vi "mhk Basic Acquisition  (no header).vi"() -> ()   [LabVIEW 2010]
uses:
  <vilib>/Utility/error.llb/DialogType.ctl
  <vilib>/DAQmx/read.llb/DAQmx Read (Analog 1D Wfm NChan NSamp).vi
  <vilib>/DAQmx/create/channels.llb/DAQmx Create Channel (AI-Voltage-Basic).vi
  <vilib>/DAQmx/configure/timing.llb/DAQmx Timing (Sample Clock).vi
  Instance          10 42Saved   mhk Basic Acquisition  (no header) .vi
  <vilib>/daqmx/miscellaneous.llb/DAQmx Fill In Error Info.vi
panel:
  in  "Prompt to Save Data?":bool caption="Enable"
  in  "Maximum Value":dbl=5.0 format="%0.2f"
  in  "Minimum Value":dbl=-5.0 format="%0.2f"
  in  "Physical Channel":tag="Dev2/ai0:1"
  in  "Rate":dbl=1000.0 caption="Sample Rate (Hz)" format="%0.2f"
  in  "Samples per Channel":i32=1000
  out "Measurement":waveform(dbl)[](graph)=[{"t0"=timestamp(3384461688.008659 s since 1904-01-01), "dt"=0.001, "Y"=array[1000 elements], "attributes"=variant("NI_ChannelName"=variant(string "Dev2/ai0"), "NI_UnitDescription"=variant(string "Volts"))}, {"t0"=timestamp(3384461688.0086718 s since 1904-01-01), "dt"=0.001, "Y"=array[1000 elements], "attributes"=variant("NI_ChannelName"=variant(string "Dev2/ai1"), "NI_UnitDescription"=variant(string "Volts"))}]
  # "Channel Parameters"
  # "Timing Parameters"
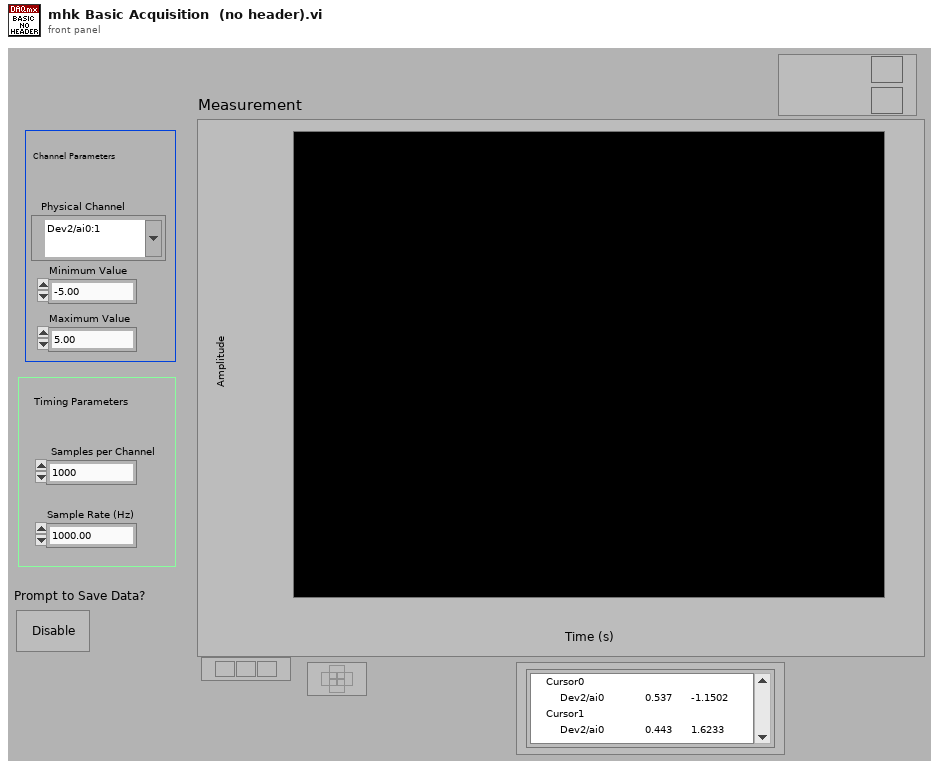
[diagram p1: front panel]
types:
  T1 = typedef "DialogType.ctl" = u16
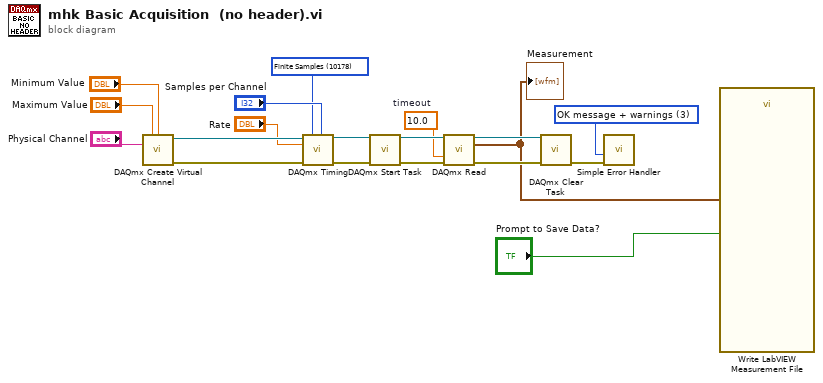
[diagram p0: block diagram]
diagram:
  w4 = T1 3 items=["no dialog", "OK message", "continue or stop message", "OK message + warnings", "continue/stop + warnings"] ("type of dialog (OK msg:1)")
  w5 = 10.0  # timeout
  w9 = 10178 items=["Finite Samples"=10178, "Continuous Samples"=10123] ("sample mode")
  n1 = call-poly <vilib>:"DAQmx Create Virtual Channel.vi"("maximum value"="Maximum Value", "minimum value"="Minimum Value", "physical channels"="Physical Channel") -> ("task out"=w13:refnum<k21>, "error out"=w17:errorcluster)  [unwired: 11 in]
  n2 = call-poly <vilib>:"DAQmx Timing.vi"("task/channels in"=w13, "sample mode"=w9, "samples per channel"="Samples per Channel", "rate"="Rate", "error in"=w17) -> ("task out"=w8:refnum<k21>, "error out"=w7:errorcluster)  [unwired: 9 in]
  n3 = call <vilib>:"DAQmx Start Task.vi"("task/channels in"=w8, "error in"=w7) -> ("task out"=w12:refnum<k21>, "error out"=w16:errorcluster)  [unwired: 12 in]
  n4 = call-poly <vilib>:"DAQmx Read.vi"("task/channels in"=w12, "timeout"=w5, "error in"=w16) -> ("task out"=w11:refnum<k21>, "data"=w2:waveform(dbl)[], "error out"=w6:errorcluster)  [unwired: 10 in]
  "Measurement" <- w2
  n5 = call <vilib>:"DAQmx Clear Task.vi"("task in"=w11, "error in"=w6) -> ("error out"=w14:errorcluster)  [unwired: 13 in]
  n6 = call <vilib>:"Simple Error Handler.vi"("type of dialog (OK msg:1)"=w4, "error in (no error)"=w14) -> ()  [unwired: 3 in, 5 out]
  n7 = call "Write LabVIEW Measurement File"("Enable"="Prompt to Save Data?", "Signals"=w2) -> ()  [unwired: 7 in, 3 out]
